vi "create_replay.vi"(4 "error in":errorcluster, 6 "Frames":string[](array[string]), 7 "Path to save":path=path "replay.json") -> (0 "error out":errorcluster)   [LabVIEW 2019]
doc: "Create a replay file from the output of a state sensor."
panel:
  out "path out":path
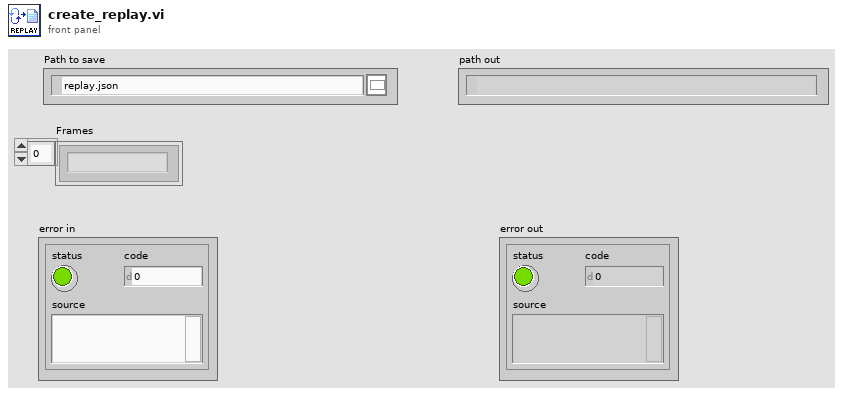
[diagram p1: front panel]
types:
  T1 = enum16{"open", "replace", "create", "open or create", "replace or create", "replace or create with confirmation"}
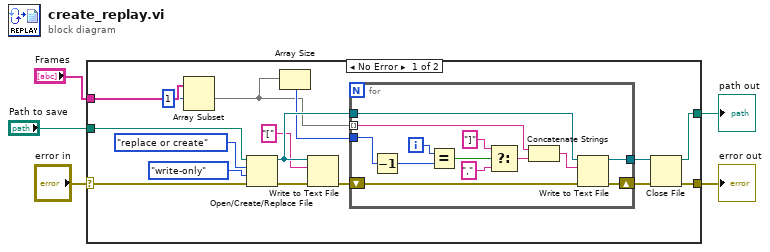
[diagram p0: block diagram]
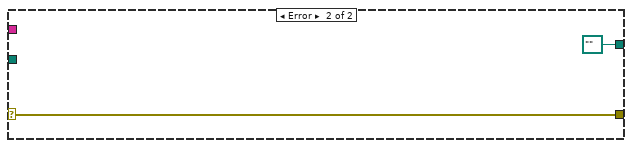
[diagram p2: hidden frame]
diagram:
  n1 = case shown="No Error" "error in" {
    selector: "error in" -> [w12 w35]
    tunnel: "Frames" -> [w8 _]
    tunnel: [w11 w35] -> w3
    tunnel: [w10 path "" ("path")] -> w2
    tunnel: "Path to save" -> [w9 _]
    frame No Error {
      n2 = Array Subset(array=w8, index=1) -> (w6:string[])  [unwired: 1 in]
      n3 = Open/Create/Replace File(file path (use dialog)=w9, error in=w12, operation (0:open)=T1."replace or create", access (0:read/write)=enum16{"read/write", "read-only", "write-only"}."write-only") -> (refnum out=w18:refnum<file>, error out=w17:errorcluster)  [unwired: 2 in, 1 out]
      n4 = Array Size(array=w6) -> (size(s)=w13:i32)
      n5 = Write to Text File(file (use dialog)=w18, text="[", error in=w17) -> (error out=w16:errorcluster)  [unwired: 1 in, 2 out]
      n6 = for {
        tunnel: w6 -> [w30] mode=indexing
        shift-right: [w34] -> w14
        shift-left: w16 -> [w31]
        tunnel: [w33] -> w21
        tunnel: w18 -> [w32]
        tunnel: w13 -> [w23]
        i -> [w24]
        n7 = Decrement(x=w23) -> (x-1=w22:i32)
        n8 = Equal?(x=w24, y=w22) -> (x = y?=w25:bool)
        n9 = Select(t="]" ("string"), s=w25, f=",") -> (s? t:f=w26:string)
        n10 = Concatenate Strings(w30, w26) -> (w29:string)
        n11 = Write to Text File(file (use dialog)=w32, text=w29, error in=w31) -> (refnum out=w33:refnum<file>, error out=w34:errorcluster)  [unwired: 1 in, 1 out]
      }
      n12 = Close File(refnum=w21, error in=w14) -> (path=w10:path, error out=w11:errorcluster)
    }
    frame Error {
    }
  }
  "error out" <- w3
  "path out" <- w2
